vi "ma_Reconstruct detected signals (CDB).vi"(9 "dt":dbl, 10 "# samples":i32, 11 "multiple tone information":T1(array[cluster]) {"detected phase (deg)" format="%.2p"; "detected amplitude" format="%.2p"; "detected frequency" format="%.2p"}) -> (2 "complex Hann spectrum":cdb[](array[numeric]), 3 "detected time array":cdb[](array[numeric]))   [LabVIEW 2020, in "NI_MAPro.lvlib"]
uses:
  NI_MAPro.lvlib
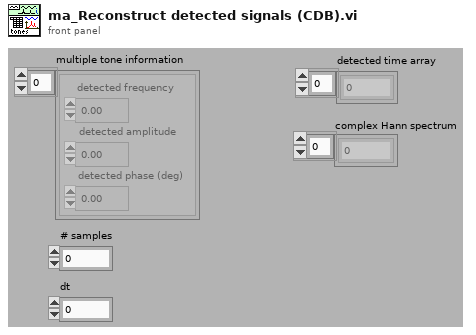
[diagram p1: front panel]
types:
  T1 = cluster{"detected frequency":dbl, "detected amplitude":dbl, "detected phase (deg)":dbl}[]
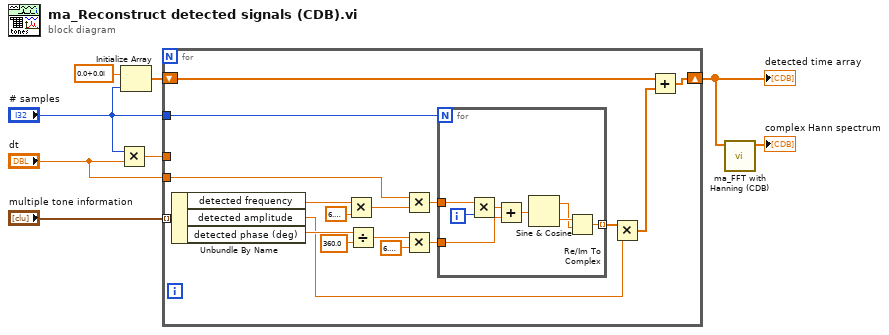
[diagram p0: block diagram]
diagram:
  n1 = Multiply(x="# samples", y="dt") -> (x*y=w7:dbl)
  n2 = Initialize Array(cdb 0.0+0.0i, "# samples") -> (w6:cdb[])
  n3 = for {
    tunnel: "multiple tone information" -> [w25] mode=indexing
    tunnel: "# samples" -> [w15]
    tunnel: w7 -> [_]
    shift-right: [w23] -> w3
    shift-left: w6 -> [w24]
    tunnel: "dt" -> [w9]
    n4 = Unbundle By Name(w25) -> ("detected frequency"=w21:dbl, "detected amplitude"=w11:dbl, "detected phase (deg)"=w16:dbl)
    n5 = Multiply(x=w21, y=6.283185307179586) -> (x*y=w20:dbl)
    n6 = Divide(x=w16, y=360.0) -> (x/y=w18:dbl)
    n7 = Multiply(x=w9, y=w20) -> (x*y=w13:dbl)
    n8 = Multiply(x=w18, y=6.283185307179586) -> (x*y=w14:dbl)
    n9 = for {
      N: w15 -> [_]
      tunnel: w14 -> [w30]
      tunnel: w13 -> [w33]
      tunnel: [w29] -> w12 mode=indexing
      i -> [w32]
      n10 = Multiply(x=w33, y=w32) -> (x*y=w31:dbl)
      n11 = Add(x=w31, y=w30) -> (x+y=w28:dbl)
      n12 = Sine & Cosine(0:w28) -> (1:w26:dbl, 2:w27:dbl)
      n13 = Re/Im To Complex(1:w26, 2:w27) -> (0:w29:cdb)
    }
    n14 = Multiply(x=w12, y=w11) -> (x*y=w10:cdb[])
    n15 = Add(x=w24, y=w10) -> (x+y=w23:cdb[])
  }
  "detected time array" <- w3
  n16 = call "ma_FFT with Hanning (CDB).vi"("time signal data"=w3) -> ("complex Hann spectrum"=→"complex Hann spectrum":cdb[])  [unwired: 10 out]
